vi "dll.midi_get_output_device_name.vi"(8 "error in (no error)":errorcluster, 10 "Device Index":i32, 11 "midi out in":refnum<class "midi out.lvclass">) -> (0 "error out":errorcluster, 2 "Name":string, 3 "midi out":refnum<class "midi out.lvclass">)   [LabVIEW 2020, in "MIDIllan.lvlib" / "midi out.lvclass"]
uses:
  midi out.lvclass
  midi out.lvclass/midi out.ctl
  MIDIllan/MIDIllan.lvlib
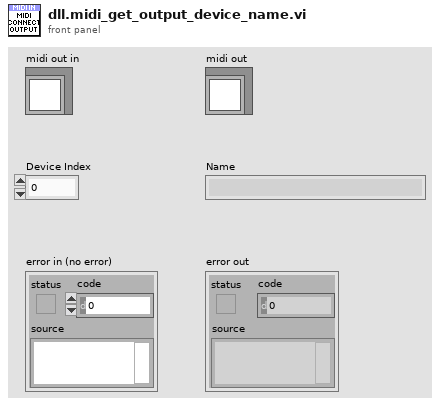
[diagram p1: front panel]
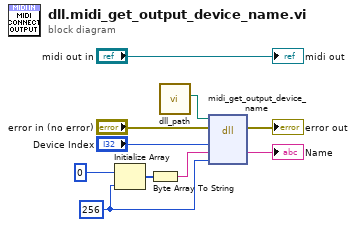
[diagram p0: block diagram]
diagram:
  w3 = 256 ("dimension size")
  n1 = Initialize Array(u8 0, w3) -> (w5:u8[])
  n2 = Byte Array To String(unsigned byte array=w5) -> (string=w4:string)
  n3 = call "dll_path.vi"() -> ("dll"=w9:path)  [unwired: 11 in]
  n4 = dll-call lib="C:/code/LabVIEW-MIDI-XPLAT/dist/TomMIDIllan_*.*" fn="midi_get_output_device_name"(path in=w9, error in="error in (no error)", "Device Index"="Device Index", "Buffer"=w4, "Buffer Sie"=w3) -> (error out=→"error out":errorcluster, "Buffer"=→"Name":string)  [unwired: 4 in, 1 out]
  "midi out" <- "midi out in"
